vi "hold trigger for permission.vi"(9 "permission":bool=TRUE, 10 "trigger":bool) -> (2 "trigger out":bool)   [LabVIEW 2010]
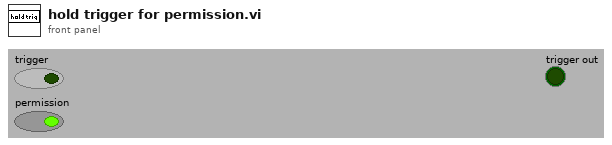
[diagram p1: front panel]
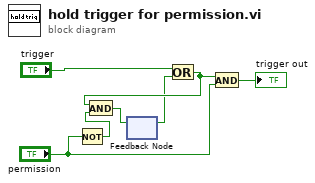
[diagram p0: block diagram]
diagram:
  n1 = Not(x="permission") -> (.not. x?=w7:bool)
  n2 = feedback #1() -> (w2:bool)  [unwired: 1 in]
  n3 = Or(x="trigger", y=w2) -> (x .or. y?=w5:bool)
  n4 = And(x=w5, y=w7) -> (x .and. y?=w4:bool)
  n5 = feedback-in #1(w4) -> ()
  n6 = And(x=w5, y="permission") -> (x .and. y?=→"trigger out":bool)
